vi "删除企业.vi"(9 "企业文件夹":path, 11 "数据库操作.i":refnum<class "数据库操作.lvclass">) -> (1 "删除企业成功？":bool, 3 "数据库操作.o":refnum<class "数据库操作.lvclass">)   [LabVIEW 2013, in "数据库操作.lvclass"]
uses:
  <vilib>/addons/database/Connection.llb/Conn Execute.vi
  <vilib>/addons/database/NI_Database_API.lvlib
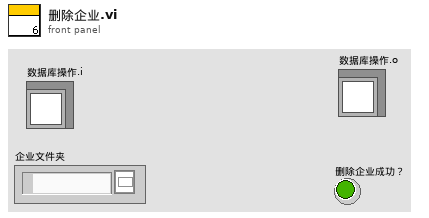
[diagram p1: front panel]
types:
  T1 = typedef "NI_Database_API.lvlib/Conn ObjectReference.ctl" = refnum<k1>
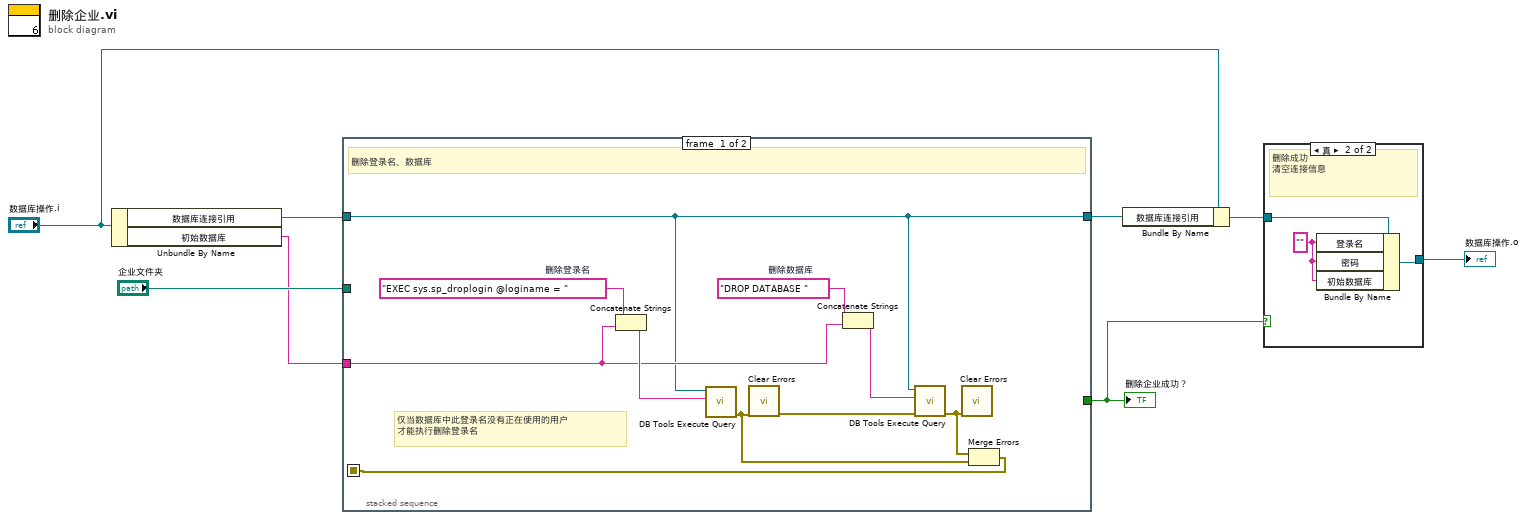
[diagram p0: block diagram]
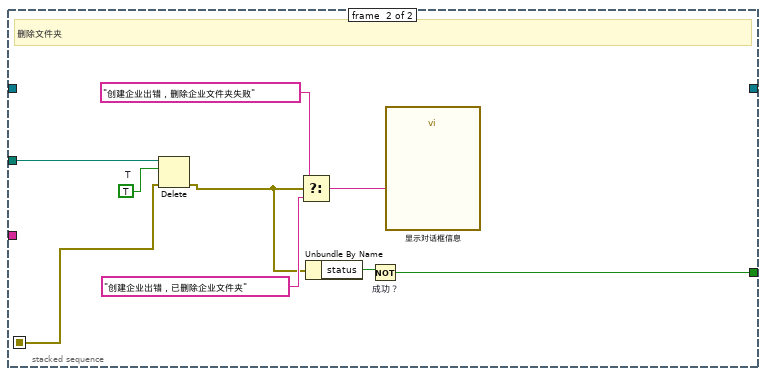
[diagram p3: hidden frame]
diagram:
  n1 = Unbundle By Name("数据库操作.i") -> ("数据库连接引用"=w8:T1, "初始数据库"=w6:string)
  n2 = stacked-sequence {
    seq-local: [w10 _] -> [_ w22]
    tunnel: w6 -> [w15 _]
    tunnel: "企业文件夹" -> [_ w26]
    tunnel: w8 -> [w9 _]
    tunnel: [_ w19] -> w3
    tunnel: [w9 _] -> w4
    frame #0 {
      w16 = "DROP DATABASE "  # 删除数据库
      w18 = "EXEC sys.sp_droplogin @loginame = "  # 删除登录名
      # "仅当数据库中此登录名没有正在使用的用户\n才能执行删除登录名"
      # "删除登录名、数据库"
      n3 = Concatenate Strings(w18, w15) -> (w17:string)
      n4 = call-poly <vilib>:"DB Tools Execute Query.vi"("SQL query"=w17, "connection reference"=w9) -> ("error out"=w11:errorcluster)  [unwired: 6 in, 1 out]
      n5 = call <vilib>:"Clear Errors.vi"("error in (no error)"=w11) -> ("error out"=w13:errorcluster)  [unwired: 6 in]
      n6 = Concatenate Strings(w16, w15) -> (w14:string)
      n7 = call-poly <vilib>:"DB Tools Execute Query.vi"("error in (no error)"=w13, "SQL query"=w14, "connection reference"=w9) -> ("error out"=w12:errorcluster)  [unwired: 5 in, 1 out]
      n8 = call <vilib>:"Clear Errors.vi"("error in (no error)"=w12) -> ()  [unwired: 6 in, 1 out]
      n9 = Merge Errors(w12, w11) -> (w10:errorcluster)
    }
    frame #1 {
      w27 = TRUE  # T
      # "删除文件夹"
      n10 = Delete(path (use dialog)=w26, entire hierarchy (F)=w27, error in=w22) -> (error out=w21:errorcluster)  [unwired: 2 in, 2 out]
      n11 = Select(t="创建企业出错，删除企业文件夹失败", s=w21, f="创建企业出错，已删除企业文件夹") -> (s? t:f=w23:string)
      n12 = Unbundle By Name(w21) -> ("status"=w20:bool)
      n13 = Not "成功？"(x=w20) -> (.not. x?=w19:bool)
      n14 = call "显示对话框信息"("Message"=w23) -> ()  [unwired: 9 in, 2 out]
    }
  }
  "删除企业成功？" <- w3
  n15 = Bundle By Name(cluster="数据库操作.i", "数据库连接引用"=w4) -> (w2:refnum<class "数据库操作.lvclass">)
  n16 = case shown="真" w3 {
    tunnel: w2 -> [w28 w30]
    tunnel: [w28 w29] -> w1
    frame False {
      # "删除失败"
    }
    frame True {
      w31 = "" ("数据库连接信息.登录名")
      # "删除成功\n清空连接信息"
      n17 = Bundle By Name(cluster=w30, "登录名"=w31, "密码"=w31, "初始数据库"=w31) -> (w29:refnum<class "数据库操作.lvclass">)
    }
  }
  "数据库操作.o" <- w1
